vi "Set ErrorCluster.vi"(8 "error in (no error)":errorcluster, 10 "ErrorCluster":errorcluster, 11 "ErrorMsg in":refnum<class "ErrorMsg.lvclass">) -> (0 "error out":errorcluster, 3 "ErrorMsg out":refnum<class "ErrorMsg.lvclass">)   [LabVIEW 2013, in "LapDog.Messaging.v3.lvlib" / "ErrorMsg.lvclass"]
doc: "Overridable accessor method for child classes to implement advanced functionality.\n\nThis method executes regardless of the error in state."
uses:
  ErrorMsg.lvclass
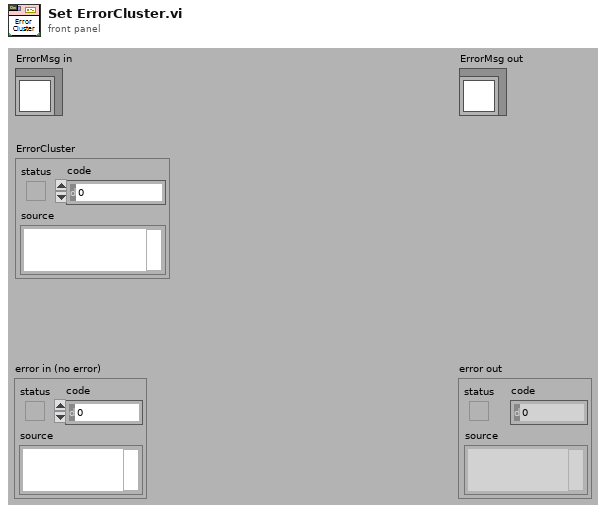
[diagram p1: front panel]
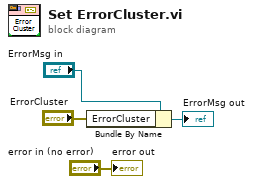
[diagram p0: block diagram]
diagram:
  n1 = Bundle By Name(cluster="ErrorMsg in", "ErrorCluster"="ErrorCluster") -> (→"ErrorMsg out":refnum<class "ErrorMsg.lvclass">)
  "error out" <- "error in (no error)"
